vi "Fetch - SParam.vi"(8 "error in":errorcluster, 11 "RFmxVNA Session in":refnum<k21>) -> (0 "error out":errorcluster, 1 "Array":cluster{"X":dbl[], "Y1":sgl[]}[](array[cluster]), 2 "Status":string, 3 "RFmxVNA Session out":refnum<k21>, 4 "S-Param Phase":dbl[][](array[numeric]), 5 "S-Param":dbl[][](array[numeric]), 6 "S-Param Magnitude":dbl[][](array[numeric]))   [LabVIEW 2023]
uses:
  <resource>/objmgr/RFmxVNA.rc
panel:
  out "SParams Results Correction State":i32
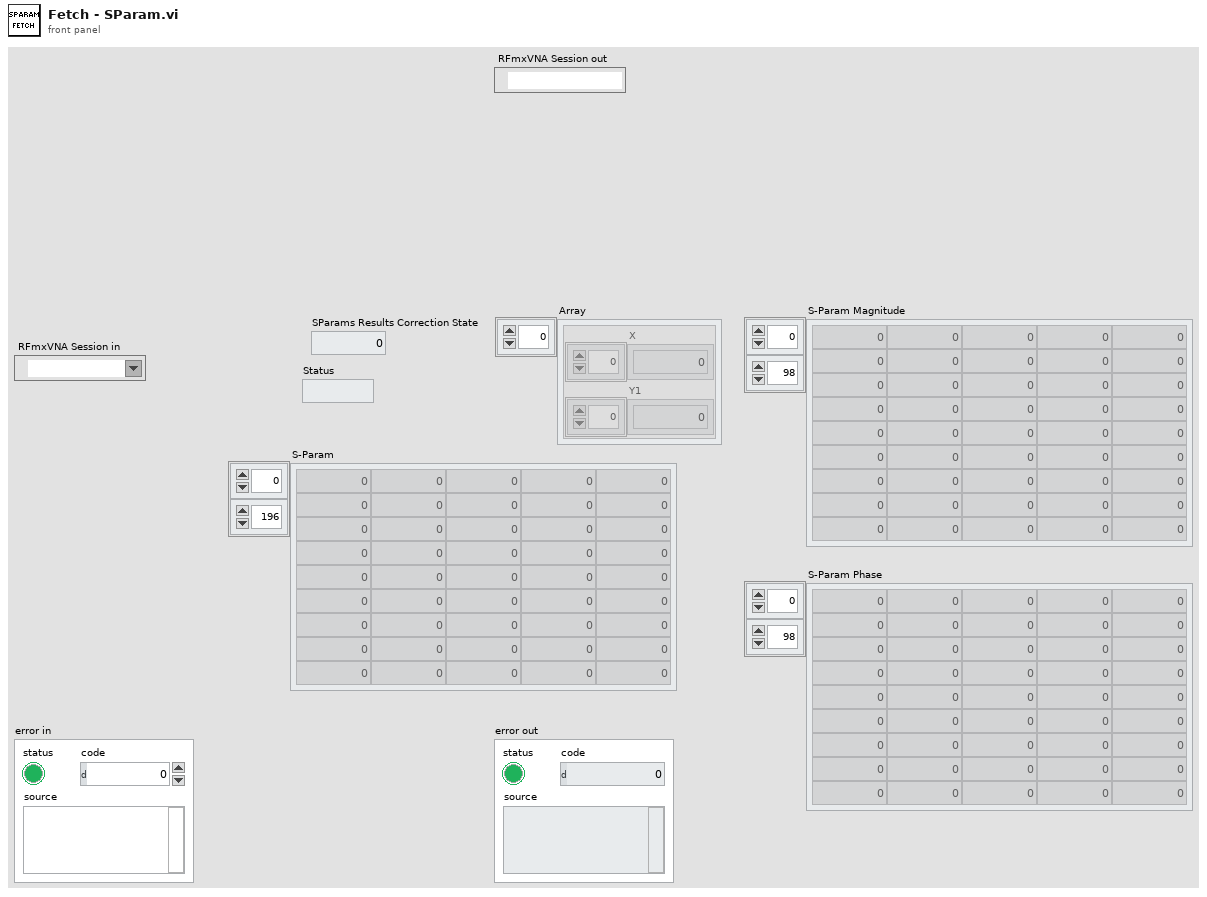
[diagram p1: front panel]
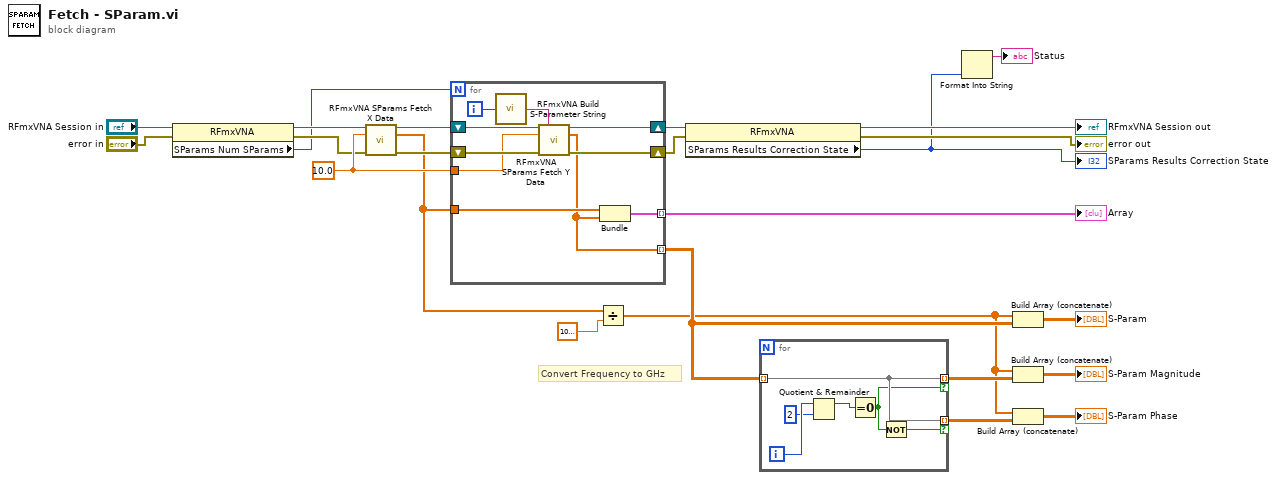
[diagram p0: block diagram]
diagram:
  w20 = 10.0 ("Timeout (s)")
  # "Convert Frequency to GHz"
  n1 = property class="RFmxVNA"(reference="RFmxVNA Session in", error in="error in") -> (reference out=w18:refnum<k21>, error out=w19:errorcluster, "SParams Num SParams"=w14:i32)
  n2 = call <vilib>:"RFmxVNA SParams Fetch X Data.vi"("Instrument Handle In"=w18, "Timeout (s)"=w20, "error in (no error)"=w19) -> ("Instrument Handle Out"=w17:refnum<k21>, "X"=w11:dbl[], "error out"=w16:errorcluster)  [unwired: 10 in]
  n3 = for {
    N: w14 -> [_]
    shift-right: [w32] -> w22
    shift-left: w16 -> [w34]
    shift-right: [w31] -> w21
    shift-left: w17 -> [w33]
    tunnel: [w30] -> w15 mode=indexing
    tunnel: w11 -> [w26]
    tunnel: w20 -> [w27]
    tunnel: [w25] -> w8 mode=indexing
    i -> [w29]
    n4 = call <vilib>:"RFmxVNA Build S-Parameter String.vi"("S-Parameter Number"=w29) -> ("Selector String Out"=w28:string)  [unwired: 14 in]
    n5 = call <vilib>:"RFmxVNA SParams Fetch Y Data.vi"("Instrument Handle In"=w33, "Selector String"=w28, "Timeout (s)"=w27, "error in (no error)"=w34) -> ("Instrument Handle Out"=w31:refnum<k21>, "Y1"=w25:sgl[], "error out"=w32:errorcluster)  [unwired: 8 in, 1 out]
    n6 = Bundle("X"=w26, "Y1"=w25) -> (w30:cluster{"X":dbl[], "Y1":sgl[]})  [unwired: 1 in]
  }
  "Array" <- w15
  n7 = Divide(x=w11, y=1000000000.0 ("Frequency (Hz)")) -> (x/y=w3:dbl[])
  n8 = property class="RFmxVNA"(reference=w21, error in=w22) -> (reference out=→"RFmxVNA Session out":refnum<k21>, error out=→"error out":errorcluster, "SParams Results Correction State"=w2:i32)
  "SParams Results Correction State" <- w2
  n9 = for {
    tunnel: w8 -> [w38] mode=indexing
    tunnel: [w38] -> w7 mode=indexing if=w36
    tunnel: [w38] -> w6 mode=indexing if=w35
    i -> [w40]
    n10 = Quotient & Remainder(x=w40, y=2) -> (x-y*floor(x/y)=w37:i32)  [unwired: 1 out]
    n11 = Equal To 0?(x=w37) -> (x = 0?=w36:bool)
    n12 = Not(x=w36) -> (.not. x?=w35:bool)
  }
  n13 = Format Into String(w2) -> (resulting string=→"Status":string)  [unwired: 3 in, 1 out]
  n14 = Build Array (concatenate)(w3, w8) -> (→"S-Param":dbl[][])
  n15 = Build Array (concatenate)(w3, w7) -> (→"S-Param Magnitude":dbl[][])
  n16 = Build Array (concatenate)(w3, w6) -> (→"S-Param Phase":dbl[][])
